vi "Modify Data format to R2_filled +split2.vi"(6 "Current set number in one current mode":i32=48, 7 "Scan number":i32=10, 8 "modified error":errorcluster, 9 "modified Data path":path, 10 "original error":errorcluster, 11 "original Data path":path) -> ()   [LabVIEW 2023]
uses:
  <vilib>/Utility/error.llb/DialogType.ctl
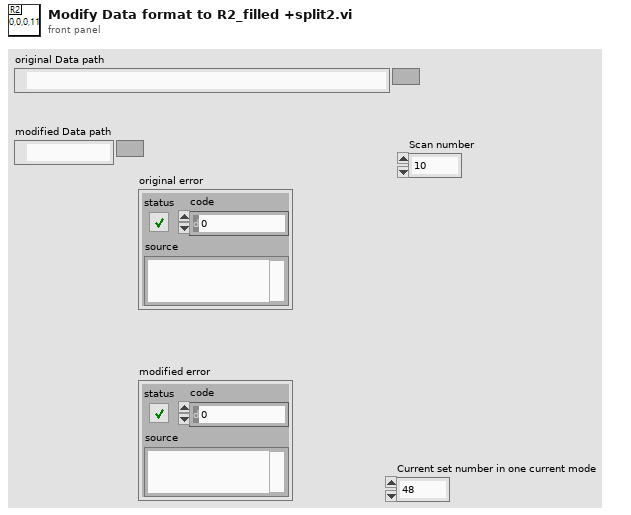
[diagram p1: front panel]
types:
  T1 = enum16{"open", "replace", "create", "open or create", "replace or create", "replace or create with confirmation"}
  T2 = typedef "DialogType.ctl" = u16
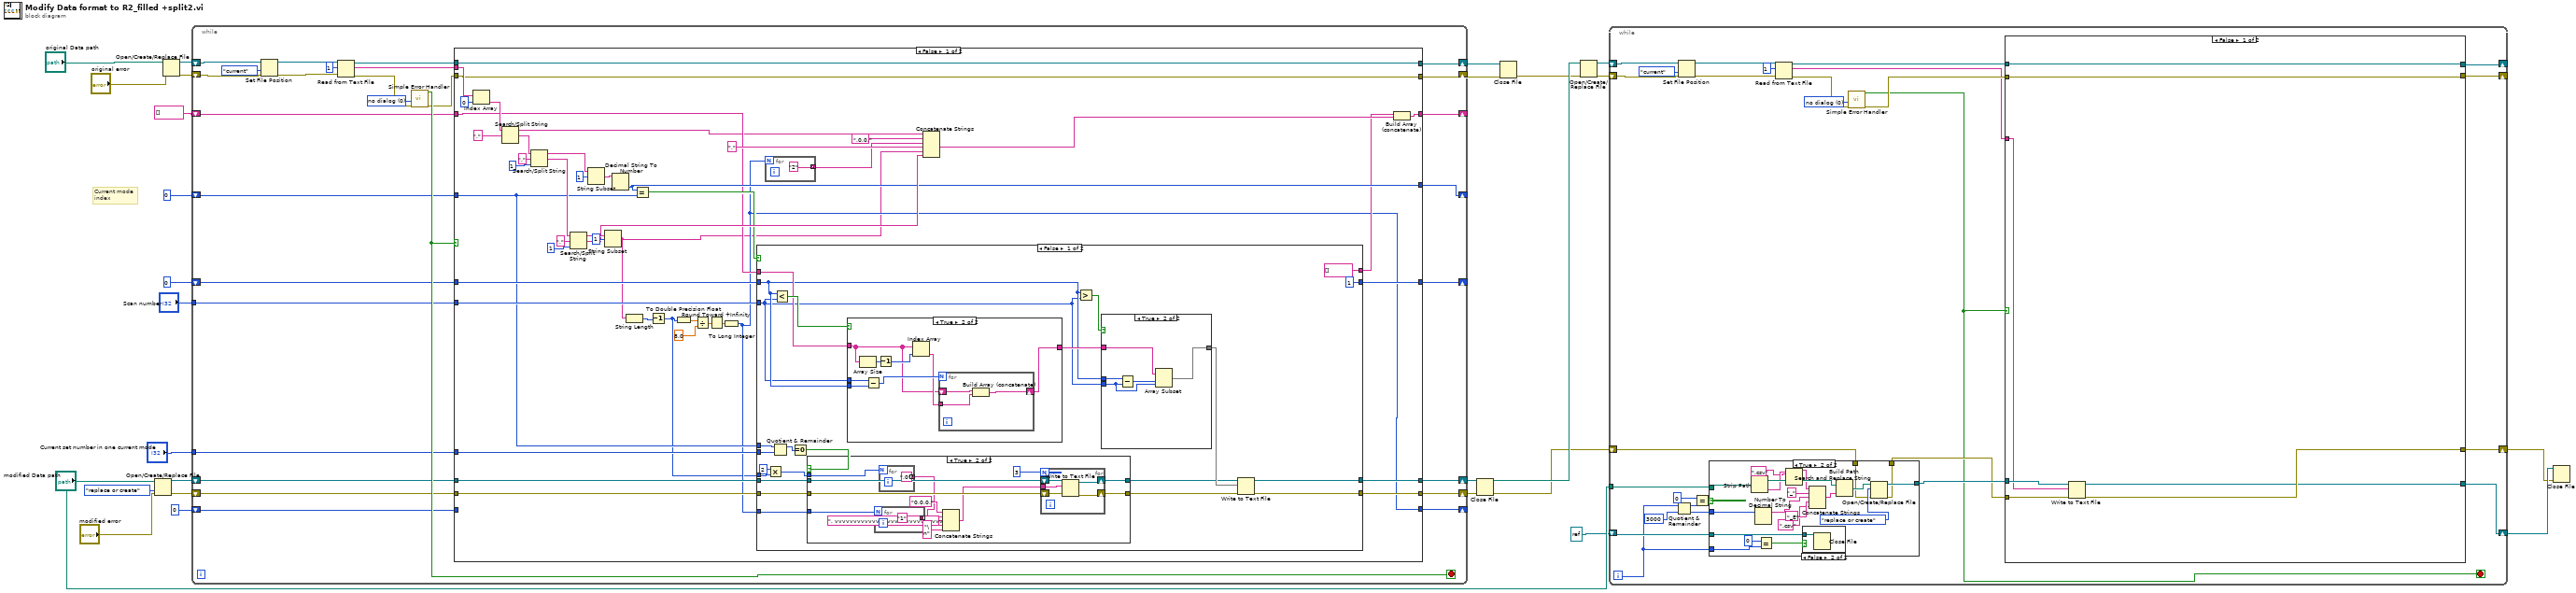
[diagram p0: block diagram]
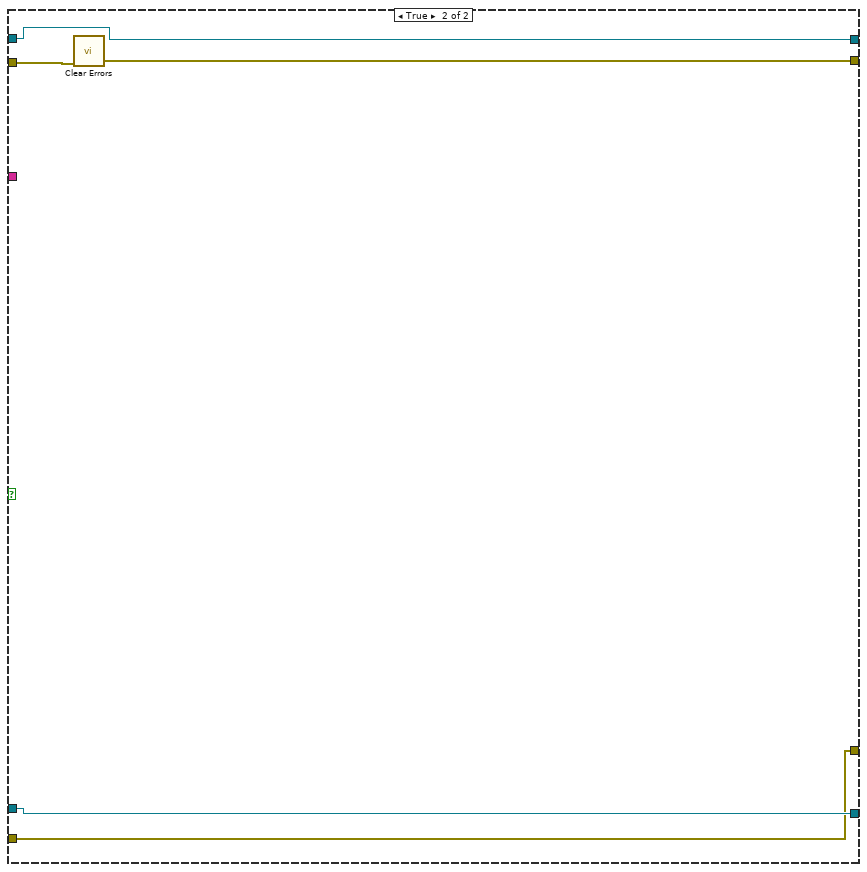
[diagram p2: hidden frame]
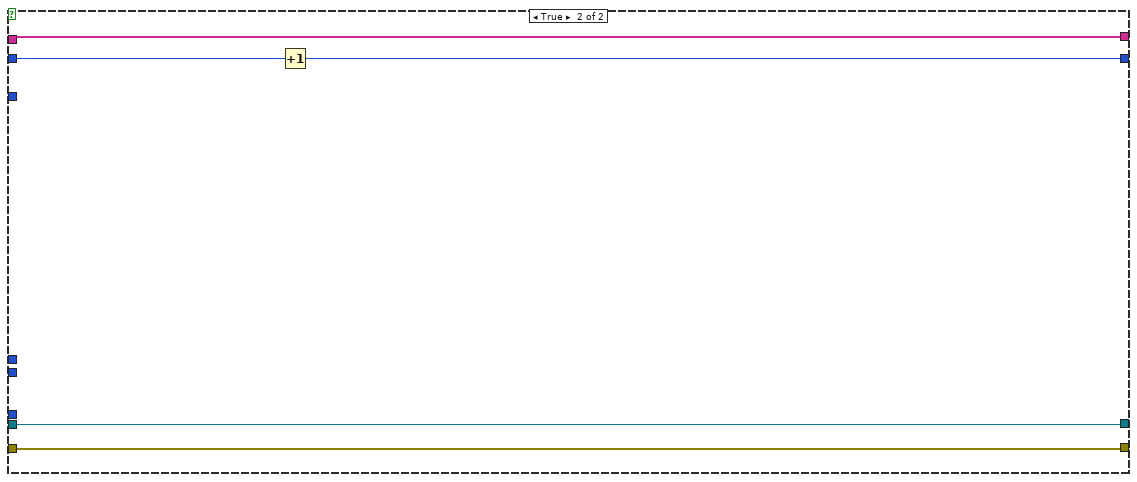
[diagram p8: hidden frame]
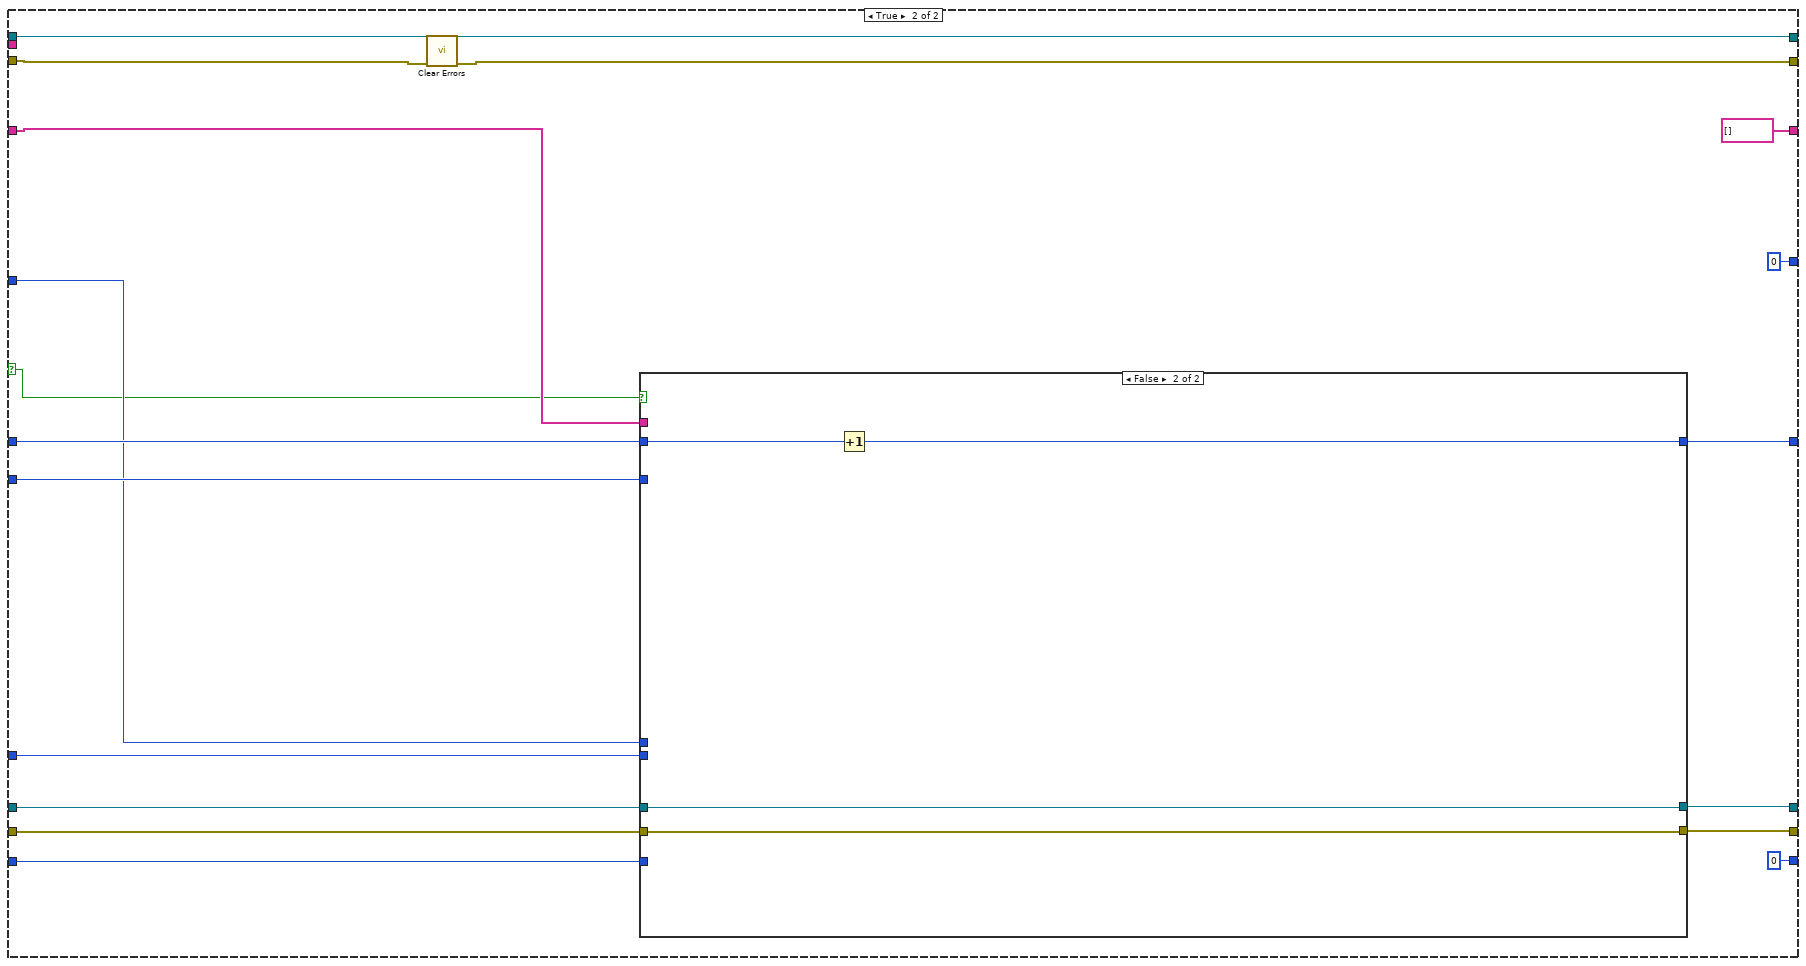
[diagram p9: hidden frame]
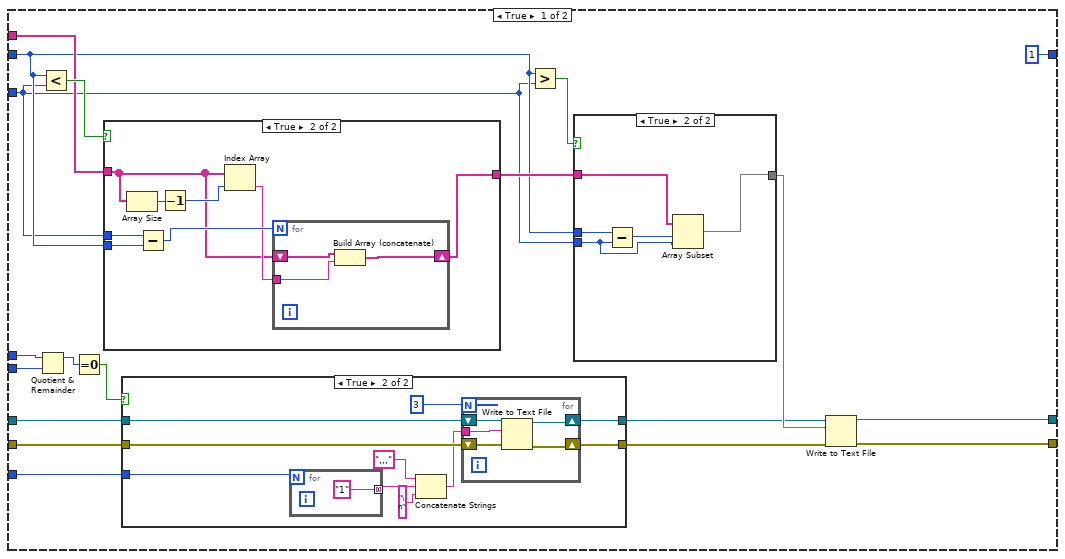
[diagram p10: hidden frame]
diagram:
  # "Current mode\nindex"
  n1 = Open/Create/Replace File(file path (use dialog)="modified Data path", error in="modified error", operation (0:open)=T1."replace or create") -> (refnum out=w24:refnum<file>, error out=w23:errorcluster)  [unwired: 3 in, 1 out]
  n2 = Open/Create/Replace File(file path (use dialog)="original Data path", error in="original error") -> (refnum out=w25:refnum<file>, error out=w26:errorcluster)  [unwired: 4 in, 1 out]
  n3 = while {
    shift-right: [w47] -> w17
    shift-left: w26 -> [w54]
    shift-right: [w46] -> w27
    shift-left: w25 -> [w45]
    shift-right: [w40] -> w19
    shift-left: w24 -> [w42]
    shift-right: [w39] -> w18
    shift-left: w23 -> [w41]
    shift-right: [w28] -> _
    shift-left: string[] [] ("element") -> [w37]
    shift-right: [w33] -> _
    shift-left: 0 ("number") -> [w36]
    shift-right: [w34] -> _
    shift-left: 0 ("number") -> [w35]
    tunnel: "Scan number" -> [w32]
    tunnel: "Current set number in one current mode" -> [w31]
    shift-right: [w30] -> _
    shift-left: 0 ("32bit integer") -> [w29]
    stop <- w51 stop-if-true
    w52 = T2 0 items=["no dialog", "OK message", "continue or stop message", "OK message + warnings", "continue/stop + warnings"] ("type of dialog (OK msg:1)")
    n4 = Set File Position(refnum=w45, from (0:start)=enum16{"start", "end", "current"}."current", error in=w54) -> (refnum out=w44:refnum<file>, error out=w43:errorcluster)  [unwired: 1 in]
    n5 = Read from Text File(file (use dialog)=w44, count=1, error in=w43) -> (refnum out=w49:refnum<file>, text=w50:string[], error out=w48:errorcluster)  [unwired: 1 in, 1 out]
    n6 = call <vilib>:"Simple Error Handler.vi"("type of dialog (OK msg:1)"=w52, "error in (no error)"=w48) -> ("error?"=w51:bool, "error out"=w38:errorcluster)  [unwired: 3 in, 3 out]
    n7 = case shown="False" w51 {
      selector: w51 -> [_ w174]
      tunnel: w50 -> [w95 _]
      tunnel: w49 -> [w93 w187]
      tunnel: w38 -> [w92 w176]
      tunnel: [w93 w187] -> w46
      tunnel: [w92 w175] -> w47
      tunnel: w42 -> [w73 w182]
      tunnel: w41 -> [w72 w181]
      tunnel: [w71 w180] -> w40
      tunnel: [w70 w179] -> w39
      tunnel: w37 -> [w75 w183]
      tunnel: w36 -> [w69 w178]
      tunnel: w35 -> [w80 w186]
      tunnel: [w79 w185] -> w34
      tunnel: [w78 0] -> w33
      tunnel: w32 -> [w76 w184]
      tunnel: w31 -> [w68 w177]
      tunnel: [w60 0] -> w30
      tunnel: w29 -> [_ w171]
      tunnel: [w59 string[] [] ("element")] -> w28
      frame False {
        n8 = Index Array(array=w95, index=0) -> (element=w91:string)
        n9 = Search/Split String(string=w91, search string/char (-)=",") -> (substring before match=w63:string, match + rest of string=w100:string)  [unwired: 1 in, 1 out]
        n10 = Search/Split String(string=w100, search string/char (-)=",", offset (0)=1) -> (substring before match=w83:string, match + rest of string=w88:string)  [unwired: 1 out]
        n11 = Search/Split String(string=w88, search string/char (-)=",", offset (0)=1) -> (substring before match=w87:string, match + rest of string=w85:string)  [unwired: 1 out]
        n12 = String Subset(string=w83, offset (0)=1) -> (substring=w82:string)  [unwired: 1 in]
        n13 = String Subset(string=w87, offset (0)=1) -> (substring=w58:string)  [unwired: 1 in]
        n14 = Decimal String To Number(string=w82) -> (number=w78:i32)  [unwired: 2 in, 1 out]
        n15 = String Length(string=w58) -> (length=w57:i32)
        n16 = Equal?(x=w78, y=w69) -> (x = y?=w81:bool)
        n17 = Decrement(x=w57) -> (x-1=w56:i32)
        n18 = To Double Precision Float(number=w56) -> (double precision float=w66:dbl)
        n19 = Divide(x=w66, y=8.0) -> (x/y=w67:dbl)
        n20 = Round Toward +Infinity(x=w67) -> (ceil(x): smallest int >= x=w64:dbl)
        n21 = To Long Integer(number=w64) -> (32bit integer=w60:i32)
        n22 = case shown="False" w81 {
          tunnel: [1 w168] -> w79
          tunnel: w80 -> [w118 w169]
          tunnel: w76 -> [w117 _]
          tunnel: w75 -> [w121 w167]
          tunnel: [string[] [] ("element") w167] -> w74
          tunnel: w73 -> [w109 w166]
          tunnel: w72 -> [w108 w165]
          tunnel: [w115 w166] -> w71
          tunnel: [w114 w165] -> w70
          tunnel: w69 -> [w113 _]
          tunnel: w68 -> [w112 _]
          tunnel: w60 -> [w105 _]
          tunnel: w56 -> [w104 _]
          frame False {
            n23 = Multiply(x=2, y=w104) -> (x*y=w102:i32)
            n24 = Quotient & Remainder(x=w113, y=w112) -> (x-y*floor(x/y)=w111:i32)  [unwired: 1 out]
            n25 = Less?(x=w118, y=w117) -> (x < y?=w122:bool)
            n26 = Equal To 0?(x=w111) -> (x = 0?=w110:bool)
            n27 = case shown="True" w110 {
              tunnel: w109 -> [w126 w136]
              tunnel: w108 -> [w125 w135]
              tunnel: [w126 w133] -> w107
              tunnel: [w125 w132] -> w106
              tunnel: w105 -> [_ w131]
              tunnel: w102 -> [_ w130]
              frame False {
              }
              frame True {
                n28 = for {
                  N: w131 -> [_]
                  tunnel: ["1" ("search string/char (-)")] -> w138 mode=concatenating
                }
                n29 = for {
                  N: w130 -> [_]
                  tunnel: [",0" ("search string/char (-)")] -> w129 mode=concatenating
                }
                n30 = Concatenate Strings("0,0,0," ("string"), w138, ", vvvvvvvvvvvvvvvvvvvvvvvvvvvvvvvv" ("string"), w129, "\n" ("string")) -> (w134:string)
                n31 = for {
                  N: 3 -> [_]
                  shift-right: [w143] -> w133
                  shift-left: w136 -> [w146]
                  tunnel: w134 -> [w144]
                  shift-right: [w142] -> w132
                  shift-left: w135 -> [w145]
                  n32 = Write to Text File(file (use dialog)=w146, text=w144, error in=w145) -> (refnum out=w143:refnum<file>, error out=w142:errorcluster)  [unwired: 1 in, 1 out]
                }
              }
            }
            n33 = case shown="True" w122 {
              tunnel: w121 -> [w153 w155]
              tunnel: w117 -> [_ w159]
              tunnel: w118 -> [_ w158]
              tunnel: [w153 w154] -> w119
              frame False {
              }
              frame True {
                n34 = Array Size(array=w155) -> (size(s)=w161:i32)
                n35 = Subtract(x=w159, y=w158) -> (x-y=w157:i32)
                n36 = Decrement(x=w161) -> (x-1=w160:i32)
                n37 = Index Array(array=w155, index=w160) -> (element=w156:string)
                n38 = for {
                  N: w157 -> [_]
                  tunnel: w156 -> [w162]
                  shift-right: [w163] -> w154
                  shift-left: w155 -> [w164]
                  n39 = Build Array (concatenate)(w164, w162) -> (w163:string[])
                }
              }
            }
            n40 = Greater?(x=w118, y=w117) -> (0:w120:bool)
            n41 = case shown="True" w120 {
              tunnel: w119 -> [w147 w151]
              tunnel: w118 -> [_ w152]
              tunnel: w117 -> [_ w149]
              tunnel: [w147 w148] -> w116
              frame False {
              }
              frame True {
                n42 = Subtract(x=w152, y=w149) -> (x-y=w150:i32)
                n43 = Array Subset(array=w151, index=w150, length=w149) -> (w148:string[])
              }
            }
            n44 = Write to Text File(file (use dialog)=w107, text=w116, error in=w106) -> (refnum out=w115:refnum<file>, error out=w114:errorcluster)  [unwired: 1 in, 1 out]
          }
          frame True {
            n45 = Increment(x=w169) -> (x+1=w168:i32)
          }
        }
        n46 = for {
          N: w60 -> [_]
          tunnel: ["2" ("search string/char (-)")] -> w61 mode=concatenating
        }
        n47 = Concatenate Strings(w63, ",0,0," ("string"), w61, "," ("string"), w58, w85) -> (w77:string)
        n48 = Build Array (concatenate)(w74, w77) -> (w59:string[])
      }
      frame True {
        n49 = call <vilib>:"Clear Errors.vi"("error in (no error)"=w176) -> ("error out"=w175:errorcluster)  [unwired: 5 in, 1 out]
        n50 = case shown="False" w174 {
          tunnel: [1 w245] -> w185
          tunnel: w186 -> [w201 w246]
          tunnel: w184 -> [w200 _]
          tunnel: w183 -> [w204 _]
          tunnel: w182 -> [w192 w244]
          tunnel: w181 -> [w191 w243]
          tunnel: [w198 w244] -> w180
          tunnel: [w197 w243] -> w179
          tunnel: w178 -> [w196 _]
          tunnel: w177 -> [w195 _]
          tunnel: w171 -> [w188 _]
          frame True {
            n51 = Quotient & Remainder(x=w196, y=w195) -> (x-y*floor(x/y)=w194:i32)  [unwired: 1 out]
            n52 = Less?(x=w201, y=w200) -> (x < y?=w205:bool)
            n53 = Equal To 0?(x=w194) -> (x = 0?=w193:bool)
            n54 = case shown="True" w205 {
              tunnel: w204 -> [w231 w233]
              tunnel: w200 -> [_ w237]
              tunnel: w201 -> [_ w236]
              tunnel: [w231 w232] -> w202
              frame False {
              }
              frame True {
                n55 = Array Size(array=w233) -> (size(s)=w239:i32)
                n56 = Subtract(x=w237, y=w236) -> (x-y=w235:i32)
                n57 = Decrement(x=w239) -> (x-1=w238:i32)
                n58 = Index Array(array=w233, index=w238) -> (element=w234:string)
                n59 = for {
                  N: w235 -> [_]
                  tunnel: w234 -> [w240]
                  shift-right: [w241] -> w232
                  shift-left: w233 -> [w242]
                  n60 = Build Array (concatenate)(w242, w240) -> (w241:string[])
                }
              }
            }
            n61 = case shown="True" w193 {
              tunnel: w192 -> [w208 w214]
              tunnel: w191 -> [w207 w213]
              tunnel: [w208 w211] -> w190
              tunnel: [w207 w210] -> w189
              tunnel: w188 -> [_ w209]
              frame False {
              }
              frame True {
                n62 = for {
                  N: w209 -> [_]
                  tunnel: ["1" ("search string/char (-)")] -> w217 mode=concatenating
                }
                n63 = Concatenate Strings(",,," ("string"), w217, "\n" ("string")) -> (w212:string)
                n64 = for {
                  N: 3 -> [_]
                  shift-right: [w221] -> w211
                  shift-left: w214 -> [w224]
                  tunnel: w212 -> [w222]
                  shift-right: [w220] -> w210
                  shift-left: w213 -> [w223]
                  n65 = Write to Text File(file (use dialog)=w224, text=w222, error in=w223) -> (refnum out=w221:refnum<file>, error out=w220:errorcluster)  [unwired: 1 in, 1 out]
                }
              }
            }
            n66 = Greater?(x=w201, y=w200) -> (0:w203:bool)
            n67 = case shown="True" w203 {
              tunnel: w202 -> [w225 w229]
              tunnel: w201 -> [_ w230]
              tunnel: w200 -> [_ w227]
              tunnel: [w225 w226] -> w199
              frame False {
              }
              frame True {
                n68 = Subtract(x=w230, y=w227) -> (x-y=w228:i32)
                n69 = Array Subset(array=w229, index=w228, length=w227) -> (w226:string[])
              }
            }
            n70 = Write to Text File(file (use dialog)=w190, text=w199, error in=w189) -> (refnum out=w198:refnum<file>, error out=w197:errorcluster)  [unwired: 1 in, 1 out]
          }
          frame False {
            n71 = Increment(x=w246) -> (x+1=w245:i32)
          }
        }
      }
    }
  }
  n72 = Close File(refnum=w19, error in=w18) -> (path=w8:path, error out=w3:errorcluster)
  n73 = Close File(refnum=w27, error in=w17) -> (error out=w4:errorcluster)  [unwired: 1 out]
  n74 = Open/Create/Replace File(file path (use dialog)=w8, error in=w4) -> (refnum out=w7:refnum<file>, error out=w9:errorcluster)  [unwired: 4 in, 1 out]
  n75 = while {
    shift-right: [w253] -> _
    shift-left: w9 -> [w272]
    shift-right: [w254] -> _
    shift-left: w7 -> [w268]
    shift-right: [w249] -> w1
    shift-left: w3 -> [w258]
    shift-right: [w248] -> w2
    shift-left: refnum<file> refnum ("refnum out") -> [w260]
    tunnel: "modified Data path" -> [w259]
    i -> [w257]
    stop <- w247 stop-if-true
    w270 = T2 0 items=["no dialog", "OK message", "continue or stop message", "OK message + warnings", "continue/stop + warnings"] ("type of dialog (OK msg:1)")
    n76 = Quotient & Remainder(x=w257, y=3000) -> (x-y*floor(x/y)=w265:i32, floor(x/y)=w262:i32)
    n77 = Set File Position(refnum=w268, from (0:start)=enum16{"start", "end", "current"}."current", error in=w272) -> (refnum out=w267:refnum<file>, error out=w266:errorcluster)  [unwired: 1 in]
    n78 = Equal?(x=0, y=w265) -> (x = y?=w263:bool)
    n79 = case shown="True" w263 {
      tunnel: w259 -> [_ w303]
      tunnel: w262 -> [_ w304]
      tunnel: [w286 w300] -> w251
      tunnel: w258 -> [w287 w299]
      tunnel: [w287 w298] -> w250
      tunnel: w260 -> [w286 w297]
      tunnel: w257 -> [_ w295]
      frame False {
      }
      frame True {
        n80 = Strip Path(path=w303) -> (stripped path=w307:path, name=w292:string)
        n81 = Number To Decimal String(number=w304) -> (decimal integer string=w288:string)  [unwired: 1 in]
        n82 = Equal?(x=0, y=w295) -> (x = y?=w293:bool)
        n83 = Search and Replace String(input string=w292, search string=".csv") -> (result string=w290:string)  [unwired: 6 in, 3 out]
        n84 = case shown="False" w293 {
          tunnel: w297 -> [_ w308]
          frame True {
          }
          frame False {
            n85 = Close File(refnum=w308) -> ()  [unwired: 1 in, 2 out]
          }
        }
        n86 = Concatenate Strings(w290, "_" ("string"), w288, "_E" ("string"), ".csv" ("string")) -> (w306:string)
        n87 = Build Path(base path=w307, name or relative path=w306) -> (appended path=w301:path)
        n88 = Open/Create/Replace File(file path (use dialog)=w301, error in=w299, operation (0:open)=T1."replace or create") -> (refnum out=w300:refnum<file>, error out=w298:errorcluster)  [unwired: 3 in, 1 out]
      }
    }
    n89 = Read from Text File(file (use dialog)=w267, count=1, error in=w266) -> (refnum out=w256:refnum<file>, text=w252:string[], error out=w269:errorcluster)  [unwired: 1 in, 1 out]
    n90 = call <vilib>:"Simple Error Handler.vi"("type of dialog (OK msg:1)"=w270, "error in (no error)"=w269) -> ("error?"=w247:bool, "error out"=w255:errorcluster)  [unwired: 3 in, 3 out]
    n91 = case shown="False" w247 {
      tunnel: w256 -> [w280 w283]
      tunnel: w255 -> [w279 w285]
      tunnel: [w280 w283] -> w254
      tunnel: [w279 w284] -> w253
      tunnel: w252 -> [w274 _]
      tunnel: w251 -> [w278 w282]
      tunnel: w250 -> [w277 w281]
      tunnel: [w276 w281] -> w249
      tunnel: [w275 w282] -> w248
      frame False {
        n92 = Write to Text File(file (use dialog)=w278, text=w274, error in=w277) -> (refnum out=w275:refnum<file>, error out=w276:errorcluster)  [unwired: 1 in, 1 out]
      }
      frame True {
        n93 = call <vilib>:"Clear Errors.vi"("error in (no error)"=w285) -> ("error out"=w284:errorcluster)  [unwired: 5 in, 1 out]
      }
    }
  }
  n94 = Close File(refnum=w2, error in=w1) -> ()  [unwired: 2 out]
